vi "Process SDIR.vi"(11 "FHPP in":refnum<class "FHPP.lvclass">) -> (3 "FHPP out":refnum<class "FHPP.lvclass">)   [LabVIEW 2022 SP3, in "FHPP.lvclass"]
uses:
  FHPP.lvclass
  FHPP.lvclass/FHPP.ctl
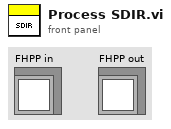
[diagram p1: front panel]
types:
  T1 = typedef "FHPP.lvclass/Setpoints.ctl" = cluster{"Vel/VelRamp (%)":u8, "Setpoint":u32}
  T2 = typedef "FHPP.lvclass/DIR.ctl" = cluster{"Relative":bool, "Control Mode":enum8{"Position", "Force", "Velocity", "Reserved"}, "Function":enum8{"Reserved", "External Input", "External Input with  Cam", "Virtual Master with Cam"}, "Function Group":enum8{"No Function", "Reserver 1", "Reserved 2", "Reserved 3"}, "Camming":bool}
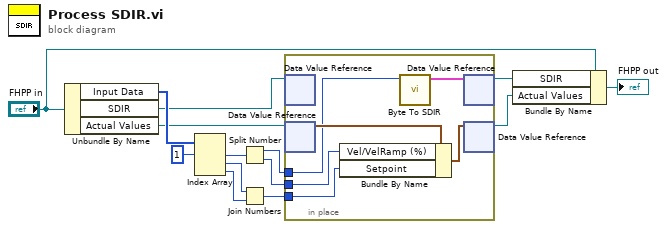
[diagram p0: block diagram]
diagram:
  n1 = Unbundle By Name("FHPP in") -> ("Input Data"=w14:u16[], "SDIR"=w5:refnum<data-value>, "Actual Values"=w9:refnum<data-value>)
  n2 = Index Array(array=w14, index #1=1 ("index")) -> (element #1=w12:u16, element #2=w11:u16, element #3=w10:u16)  [unwired: 2 in]
  n3 = Split Number(x=w12) -> (hi(x)=w6:u8, lo(x)=w7:u8)
  n4 = Join Numbers(hi=w11, lo=w10) -> ((hi.lo)=w8:u32)
  n5 = in-place {
    in-place-border: w8 -> [w19]
    in-place-border: w7 -> [w18]
    in-place-border: w6 -> [w16]
    n6 = in-place-dvr #1(w5) -> ()  [unwired: 2 out]
    n7 = in-place-dvr #2(w9) -> (w20:T1)  [unwired: 1 out]
    n8 = Bundle By Name(cluster=w20, "Vel/VelRamp (%)"=w18, "Setpoint"=w19) -> (w15:T1)
    n9 = call "Byte To SDIR.vi"("Numeric"=w16) -> ("DIR"=w17:T2)  [unwired: 10 in]
    n10 = in-place-dvr #1(w17) -> (w2:refnum<data-value>)  [unwired: 1 out]
    n11 = in-place-dvr #2(w15) -> (w1:refnum<data-value>)  [unwired: 1 out]
  }
  n12 = Bundle By Name(cluster="FHPP in", "SDIR"=w2, "Actual Values"=w1) -> (→"FHPP out":refnum<class "FHPP.lvclass">)
